vi "ReadREPL.vi"(8 "error in (no error)":errorcluster, 11 "VISA Refnum in":refnum<visa-resource-name>) -> (0 "error out":errorcluster, 1 "bytes read":u32, 2 "String":string, 3 "VISA Refnum out":refnum<visa-resource-name>)   [LabVIEW 2020]
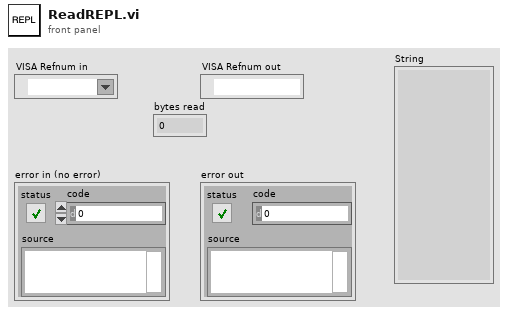
[diagram p1: front panel]
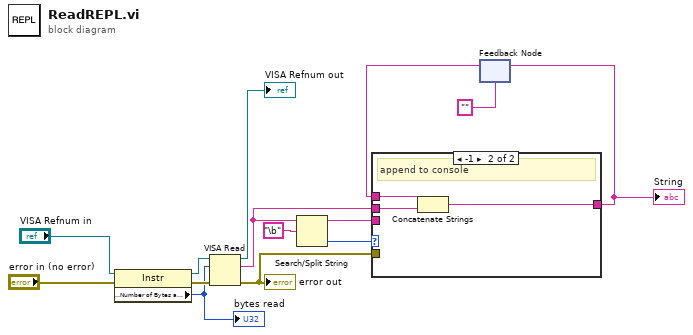
[diagram p0: block diagram]
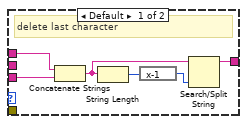
[diagram p2: hidden frame]
diagram:
  n1 = property class="Instr"(reference="VISA Refnum in", error in="error in (no error)") -> (reference out=w5:refnum<visa-resource-name>, error out=w4:errorcluster, "Serial Settings:Number of Bytes at Serial Port"=w3:u32)
  "bytes read" <- w3
  n2 = VISA Read(VISA resource name=w5, byte count=w3, error in (no error)=w4) -> (VISA resource name out=→"VISA Refnum out":refnum<visa-resource-name>, read buffer=w6:string, error out=w13:errorcluster)  [unwired: 1 out]
  "error out" <- w13
  n3 = Search/Split String(string=w6, search string/char (-)="\b") -> (substring before match=w8:string, offset of match=w7:i32)  [unwired: 1 in, 1 out]
  n4 = feedback #1("") -> (w14:string)
  n5 = case shown="-1" w7 {
    tunnel: w8 -> [w15 _]
    tunnel: w6 -> [_ w21]
    tunnel: [w17 w23] -> w1
    tunnel: w13 -> [_ _]
    tunnel: w14 -> [w16 w22]
    frame Default {
      # "delete last character"
      n6 = Concatenate Strings(w16, w15) -> (w18:string)
      n7 = String Length(string=w18) -> (length=w19:i32)
      n8 = expression code="x-1"(w19) -> (w20:i32)
      n9 = Search/Split String(string=w18, offset (0)=w20) -> (substring before match=w17:string)  [unwired: 1 in, 2 out]
    }
    frame -1 {
      # "append to console"
      n10 = Concatenate Strings(w22, w21) -> (w23:string)
    }
  }
  "String" <- w1
  n11 = feedback-in #1(w1) -> ()
